vi "ts_tree_clear.vi"(8 "error in (no error)":errorcluster, 11 "Tree.in":refnum<vi>) -> (0 "error out":errorcluster, 3 "Tree.out":refnum<vi>)   [LabVIEW 2015]
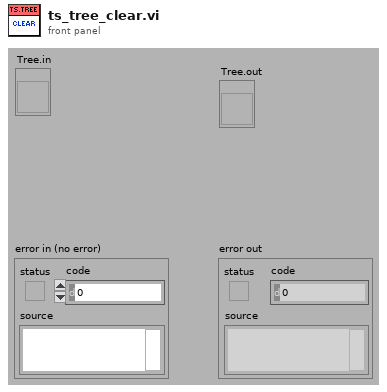
[diagram p1: front panel]
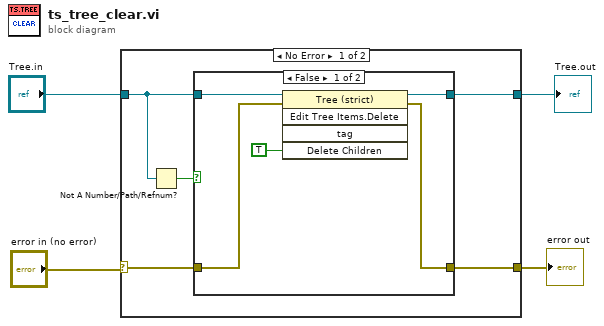
[diagram p0: block diagram]
diagram:
  n1 = case shown="No Error" "error in (no error)" {
    selector: "error in (no error)" -> [w8 w17]
    tunnel: "Tree.in" -> [w5 w18]
    tunnel: [w9 w18] -> w2
    tunnel: [w7 w17] -> w1
    frame No Error {
      n2 = Not A Number/Path/Refnum?(number/path/refnum=w5) -> (NaN/Path/Refnum?=w6:bool)
      n3 = case shown="False" w6 {
        tunnel: w5 -> [w13 w16]
        tunnel: [w12 w16] -> w9
        tunnel: w8 -> [w11 w15]
        tunnel: [w10 w15] -> w7
        frame False {
          n4 = invoke class="Tree (strict)" method="Edit Tree Items.Delete"(reference=w13, error in=w11, "Delete Children"=TRUE ("Delete Children?")) -> (reference out=w12:refnum<vi>, error out=w10:errorcluster)  [unwired: 2 in, 3 out]
        }
        frame True {
        }
      }
    }
    frame Error {
    }
  }
  "Tree.out" <- w2
  "error out" <- w1
